vi "main.vi"() -> ()   [LabVIEW 2023]
panel:
  out "error out":errorcluster
  in  "error in (no error)":errorcluster
  in  "wait":bool
  in  "Stop":bool
  in  "Run Popup":bool
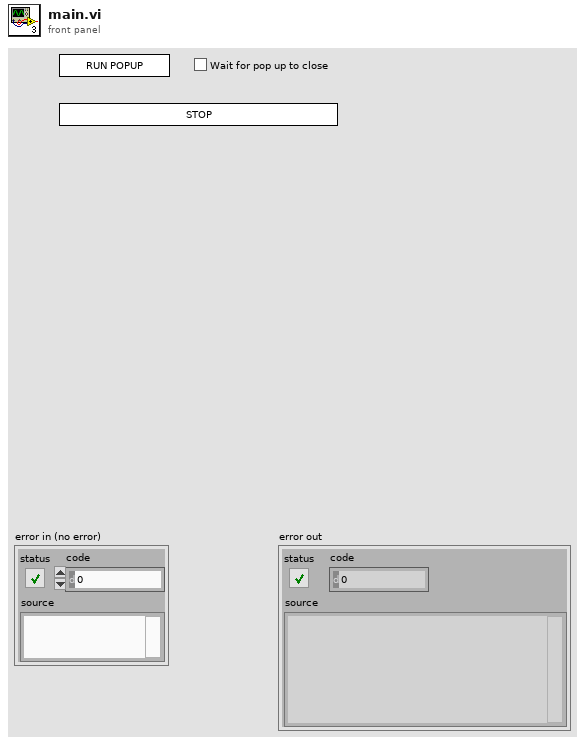
[diagram p1: front panel]
types:
  T1 = enum32{"Invalid", "Default", "Floating", "Floating/Auto-Hide", "Modal"}
  T2 = enum32{"Bad", "Idle", "Run top level", "Running"}
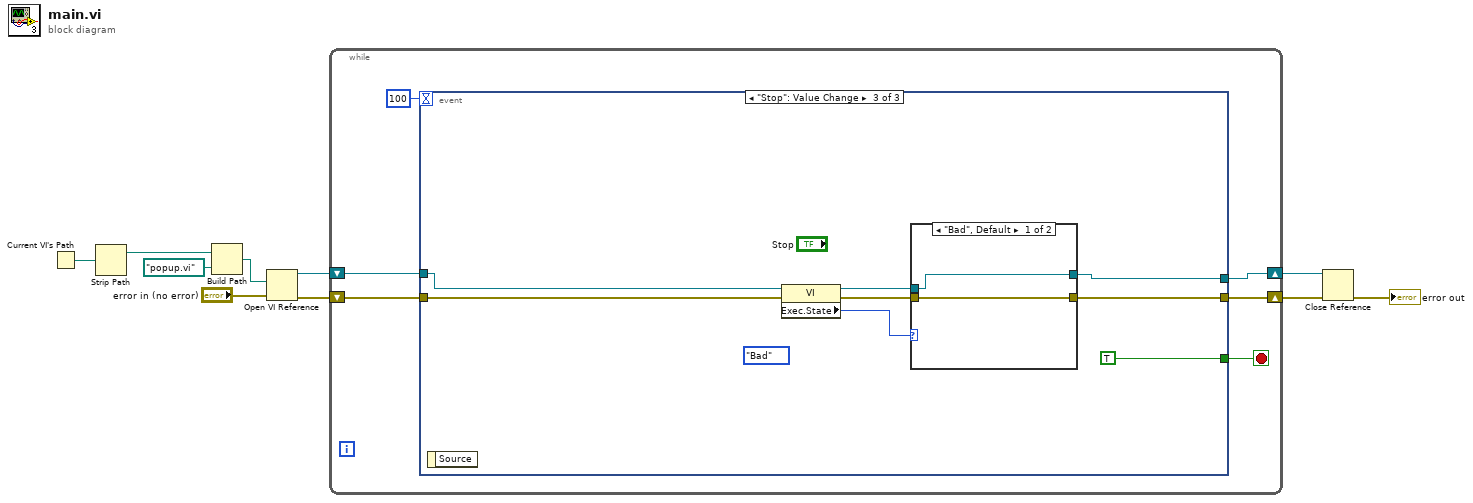
[diagram p0: block diagram]
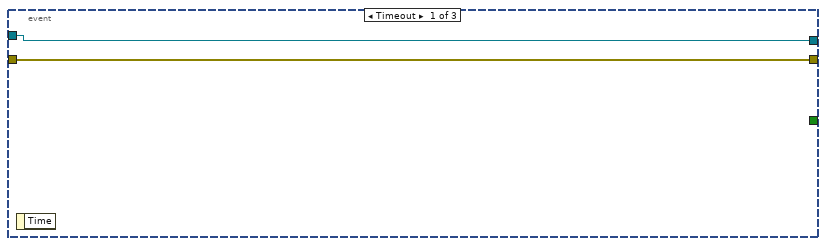
[diagram p2: hidden frame]
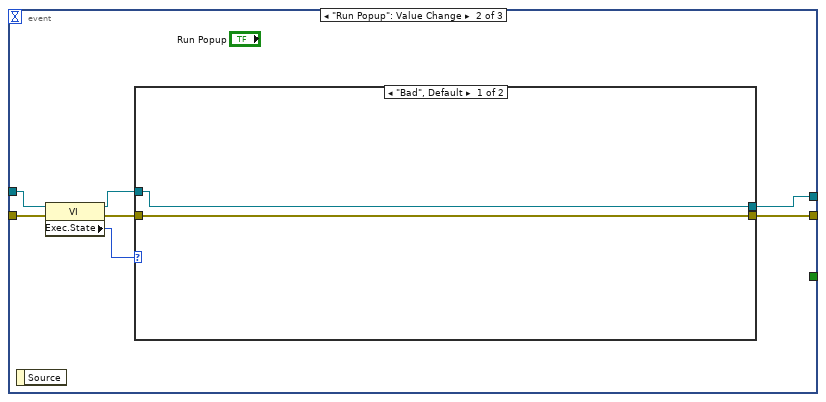
[diagram p3: hidden frame]
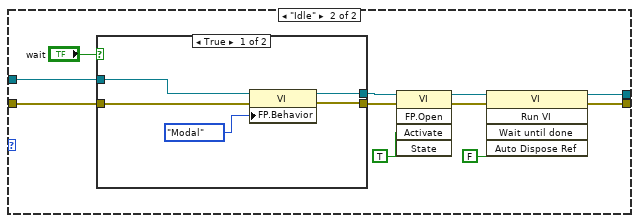
[diagram p4: hidden frame]
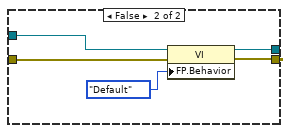
[diagram p5: hidden frame]
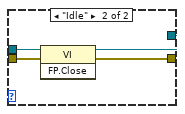
[diagram p6: hidden frame]
diagram:
  n1 = Current VI's Path() -> (path=w7:path)
  n2 = Strip Path(path=w7) -> (stripped path=w6:path)  [unwired: 1 out]
  n3 = Build Path(base path=w6, name or relative path=path "popup.vi") -> (appended path=w8:path)
  n4 = Open VI Reference(vi path=w8, error in (no error)="error in (no error)") -> (vi reference=w4:refnum<vi>, error out=w1:errorcluster)  [unwired: 4 in]
  n5 = while {
    shift-right: [w15] -> w9
    shift-left: w1 -> [w16]
    shift-right: [w11] -> w2
    shift-left: w4 -> [w12]
    stop <- w14 stop-if-true
    n6 = event shown="[2] \"Stop\": Value Change" {
      selector: _ -> [_ _ _]
      dyn-events: _ -> [_ _ _]
      timeout: 100 -> [_ _ _]
      tunnel: w16 -> [w18 w23 w56]
      tunnel: [w18 w25 w50] -> w15
      tunnel: [_ _ TRUE] -> w14
      tunnel: w12 -> [w17 w21 w51]
      tunnel: [w17 w24 w49] -> w11
      event Timeout {
        n7 = event-data() -> ()  [unwired: 1 in, 1 out]
      }
      event "Run Popup": Value Change {
        n8 = event-data() -> ()  [unwired: 1 in, 1 out]
        n9 = property class="VI"(reference=w21, error in=w23) -> (reference out=w20:refnum<vi>, error out=w22:errorcluster, "Exec.State"=w19:T2)
        n10 = case shown="\"Bad\", Default" w19 {
          tunnel: [w26 w38] -> w25
          tunnel: [w27 w33] -> w24
          tunnel: w22 -> [w26 w31]
          tunnel: w20 -> [w27 w29]
          frame "Bad", Default {
          }
          frame "Idle" {
            n11 = case shown="True" "wait" {
              tunnel: w31 -> [w42 w47]
              tunnel: w29 -> [w43 w48]
              tunnel: [w40 w45] -> w32
              tunnel: [w39 w44] -> w28
              frame True {
                n12 = property class="VI"(reference=w43, error in=w42, "FP.Behavior"=T1."Modal" ("Front Panel Window:Behavior")) -> (reference out=w39:refnum<vi>, error out=w40:errorcluster)
              }
              frame False {
                n13 = property class="VI"(reference=w48, error in=w47, "FP.Behavior"=T1."Default" ("Front Panel Window:Behavior")) -> (reference out=w44:refnum<vi>, error out=w45:errorcluster)
              }
            }
            n14 = invoke class="VI" method="FP.Open"(reference=w28, error in=w32, "Activate"=TRUE ("Activate?")) -> (reference out=w37:refnum<vi>, error out=w36:errorcluster)  [unwired: 2 in, 3 out]
            n15 = invoke class="VI" method="Run VI"(reference=w37, error in=w36, "Wait until done"=FALSE ("Wait Until Done")) -> (reference out=w33:refnum<vi>, error out=w38:errorcluster)  [unwired: 2 in, 3 out]
          }
        }
      }
      event "Stop": Value Change {
        (unwired) T2."Bad" ("Execution:State")
        n16 = event-data() -> ()  [unwired: 1 in, 1 out]
        n17 = property class="VI"(reference=w51, error in=w56) -> (reference out=w55:refnum<vi>, error out=w54:errorcluster, "Exec.State"=w53:T2)
        n18 = case shown="\"Bad\", Default" w53 {
          tunnel: w54 -> [w58 w62]
          tunnel: w55 -> [w57 w61]
          tunnel: [w58 w60] -> w50
          tunnel: [w57 w59] -> w49
          frame "Bad", Default {
          }
          frame "Idle" {
            n19 = invoke class="VI" method="FP.Close"(reference=w61, error in=w62) -> (reference out=w59:refnum<vi>, error out=w60:errorcluster)  [unwired: 1 in, 1 out]
          }
        }
      }
    }
  }
  n20 = Close Reference(reference=w2, error in (no error)=w9) -> (error out=→"error out":errorcluster)
